vi "VITester_Provider_OnCommand.vi"(10 "Command ID":string, 11 "Items Array":T1[](array[typedef])) -> ()   [LabVIEW 2013]
uses:
  <resource>/Framework/Providers/vitester-src/Support/VITester Project Item Ref.ctl
panel:
  out "error out":errorcluster
  in  "error in":errorcluster
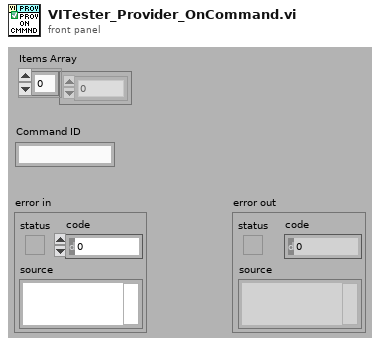
[diagram p1: front panel]
types:
  T1 = typedef "VITester Project Item Ref.ctl" = u64
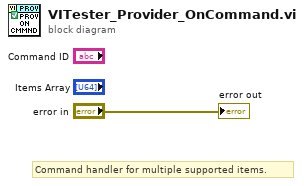
[diagram p0: block diagram]
diagram:
  # "Command handler for multiple supported items."
  "error out" <- "error in"
